vi "Launcher.vi"   [LabVIEW 2009]
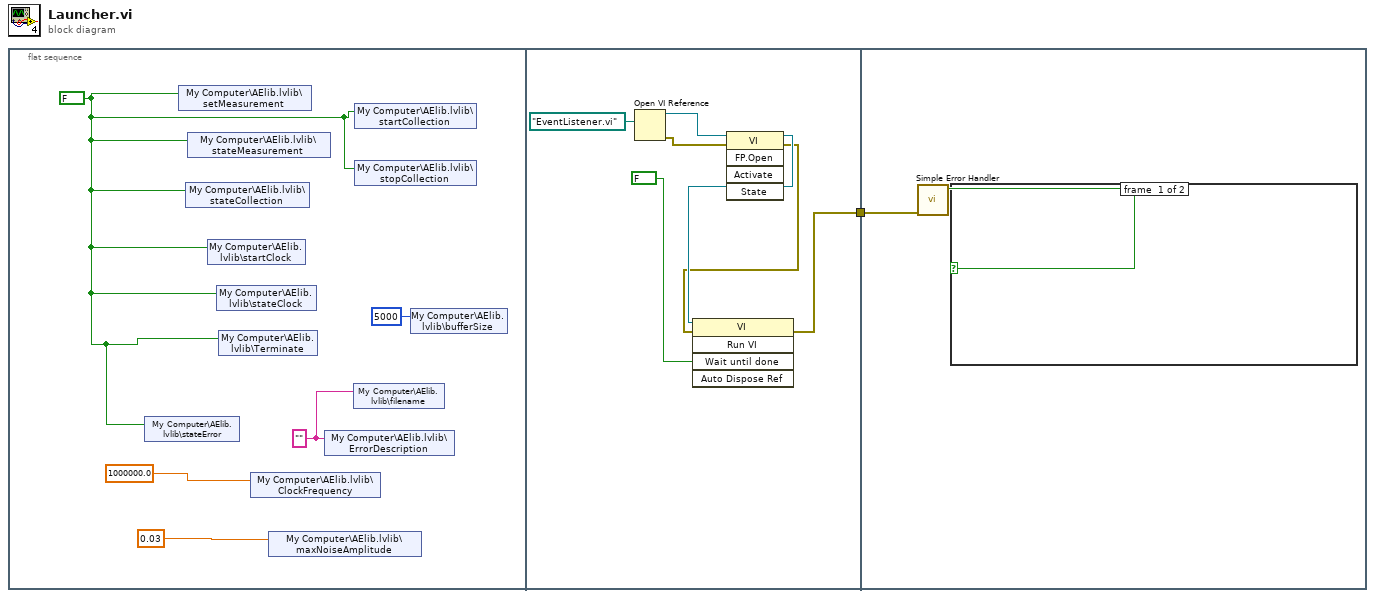
[diagram p0: block diagram]
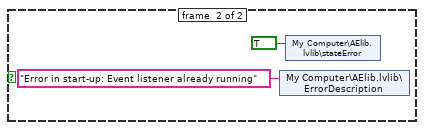
[diagram p2: hidden frame]
diagram:
  n1 = flat-sequence {
    tunnel: [w11] -> w1
    tunnel: w1 -> [w15]
    frame #0 {
      w3 = ""
      w5 = FALSE
      n2 = shared-variable "My Computer\\AElib.lvlib\\stateError"(w5) -> ()  [unwired: 1 in, 1 out]
      n3 = shared-variable "My Computer\\AElib.lvlib\\setMeasurement"(w5) -> ()  [unwired: 1 in, 1 out]
      n4 = shared-variable "My Computer\\AElib.lvlib\\stateCollection"(w5) -> ()  [unwired: 1 in, 1 out]
      n5 = shared-variable "My Computer\\AElib.lvlib\\stateMeasurement"(w5) -> ()  [unwired: 1 in, 1 out]
      n6 = shared-variable "My Computer\\AElib.lvlib\\startClock"(w5) -> ()  [unwired: 1 in, 1 out]
      n7 = shared-variable "My Computer\\AElib.lvlib\\stateClock"(w5) -> ()  [unwired: 1 in, 1 out]
      n8 = shared-variable "My Computer\\AElib.lvlib\\Terminate"(w5) -> ()  [unwired: 1 in, 1 out]
      n9 = shared-variable "My Computer\\AElib.lvlib\\ClockFrequency"(1000000.0 ("ClockFrequency")) -> ()  [unwired: 1 in, 1 out]
      n10 = shared-variable "My Computer\\AElib.lvlib\\maxNoiseAmplitude"(0.03 ("maxNoiseAmplitude")) -> ()  [unwired: 1 in, 1 out]
      n11 = shared-variable "My Computer\\AElib.lvlib\\ErrorDescription"(w3) -> ()  [unwired: 1 in, 1 out]
      n12 = shared-variable "My Computer\\AElib.lvlib\\filename"(w3) -> ()  [unwired: 1 in, 1 out]
      n13 = shared-variable "My Computer\\AElib.lvlib\\startCollection"(w5) -> ()  [unwired: 1 in, 1 out]
      n14 = shared-variable "My Computer\\AElib.lvlib\\stopCollection"(w5) -> ()  [unwired: 1 in, 1 out]
      n15 = shared-variable "My Computer\\AElib.lvlib\\bufferSize"(i16 5000 ("bufferSize")) -> ()  [unwired: 1 in, 1 out]
    }
    frame #1 {
      n16 = Open VI Reference(vi path=path "EventListener.vi") -> (vi reference=w10:refnum<vi>, error out=w8:errorcluster)  [unwired: 5 in]
      n17 = invoke class="VI" method="FP.Open"(reference=w10, error in=w8) -> (reference out=w9:refnum<vi>, error out=w7:errorcluster)  [unwired: 3 in, 3 out]
      n18 = invoke class="VI" method="Run VI"(reference=w9, error in=w7, "Wait until done"=FALSE) -> (error out=w11:errorcluster)  [unwired: 2 in, 4 out]
    }
    frame #2 {
      n19 = call <vilib>:"Simple Error Handler.vi"("error in (no error)"=w15) -> ("error?"=w14:bool)  [unwired: 4 in, 4 out]
      n20 = case shown="True" w14 {
        frame #0 {
        }
        frame #1 {
          n21 = shared-variable "My Computer\\AElib.lvlib\\ErrorDescription"("Error in start-up: Event listener already running" ("ErrorDescription")) -> ()  [unwired: 1 in, 1 out]
          n22 = shared-variable "My Computer\\AElib.lvlib\\stateError"(TRUE ("stateError")) -> ()  [unwired: 1 in, 1 out]
        }
      }
    }
  }
